vi "单个流程读取.vi"(7 "工作状态":u16, 8 "error in (no error)":errorcluster caption="错误输入（无错误）", 9 "量程":u16(ring) items=["低量程", "高量程"], 10 "测量模式":u16(ring) items=["跨度核查", "水样测量", "零点核查", "标样核查", "加标回收", "快捷测试", "空白校准", "标样校准"], 11 "测量参数":u16(ring) items=["总氮"=2, "总磷"=1, "氨氮"=3, "COD"=22]) -> (0 "error out":errorcluster, 3 "数组 2":T1(array[cluster]) {"port" format="%08x"})   [LabVIEW 2016, in "斯坦道氟化物.lvlib"]
uses:
  <vilib>/Plasmionique/MB Master/MB Master.lvlib
panel:
  out "数值":i32
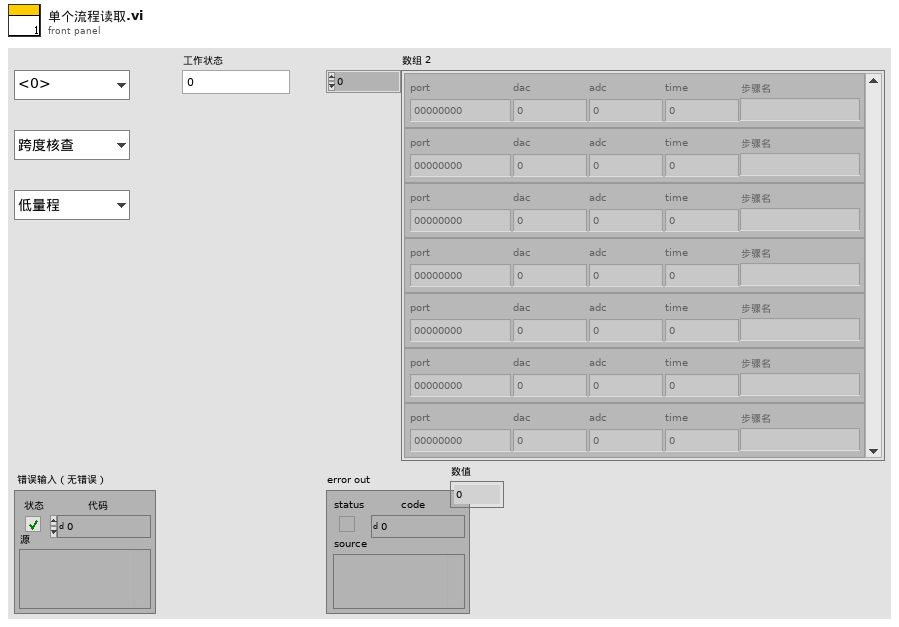
[diagram p1: front panel]
types:
  T1 = cluster{"port":i32, "dac":u8, "adc":u8, "time":u16, "步骤名":string}[]
  T2 = cluster{"port":i32, "dac":u8, "adc":u8, "time":u16, "步骤名":string}
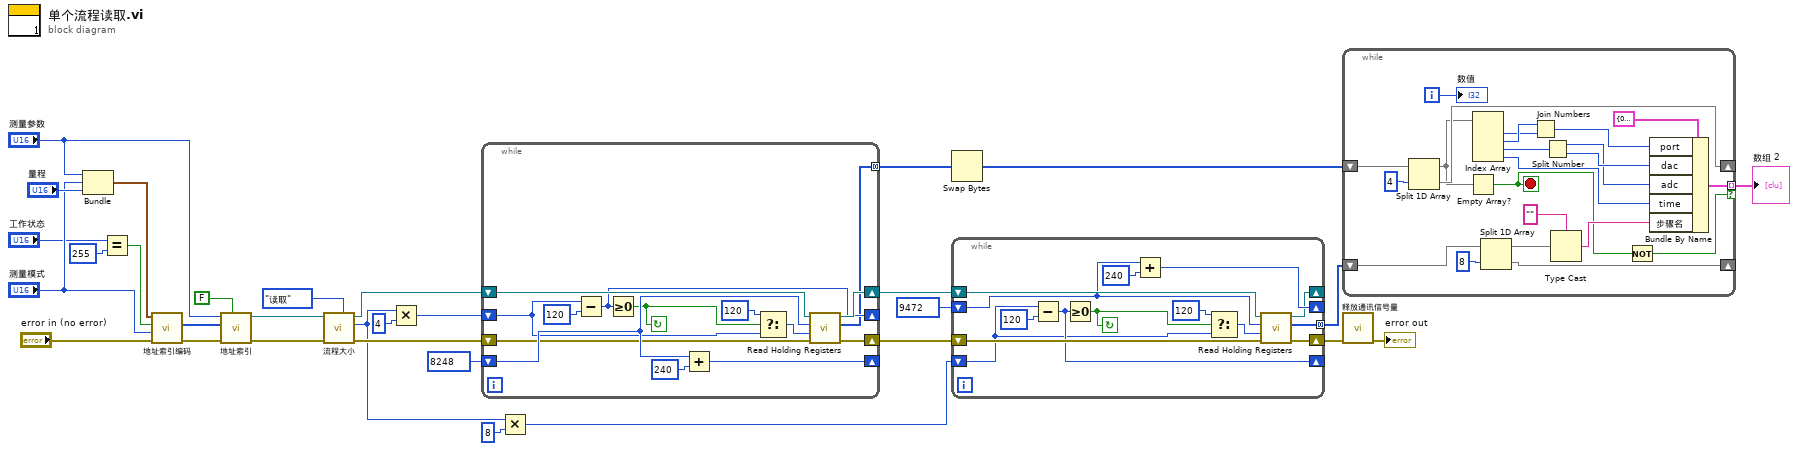
[diagram p0: block diagram]
diagram:
  n1 = Bundle("测量参数"="测量参数", "测量模式"="测量模式", "量程"="量程") -> (w26:cluster{"测量参数":u16, "测量模式":u16, "量程":u16})  [unwired: 1 in]
  n2 = Equal?(x="工作状态", y=255) -> (x = y?=w2:bool)
  n3 = call "地址索引编码.vi"("error in (no error)"="error in (no error)", "简易流程Id"="测量模式", "是否是简易流程"=w2, "参数簇"=w26) -> ("error out"=w24:errorcluster, "数组"=w25:u16[])  [unwired: 6 in]
  n4 = call "地址索引.vi"("4.2写公式？"=FALSE ("写流程？"), "error in (no error)"=w24, "values"=w25, "测量参数"="测量参数") -> ("error out"=w30:errorcluster, "MB session out"=w29:refnum<class "MB_Master.lvclass">)  [unwired: 6 in]
  n5 = call "流程大小.vi"("功能"=enum16{"写入", "读取"}."读取", "error in (no error)"=w30, "MB session in"=w29) -> ("error out"=w11:errorcluster, "大小读取"=w9:i32, "MB session out"=w10:refnum<class "MB_Master.lvclass">)  [unwired: 6 in]
  n6 = Multiply(x=w9, y=4) -> (x*y=w22:i32)
  n7 = while {
    shift-right: [w44] -> _
    shift-left: u16 8248 ("starting address") -> [w41]
    shift-right: [w43] -> w17
    shift-left: w10 -> [w42]
    shift-right: [w40] -> w16
    shift-left: w11 -> [w39]
    shift-right: [w37] -> _
    shift-left: w22 -> [w36]
    tunnel: [w32] -> w14 mode=concatenating
    stop <- w34 continue-if-true
    n8 = Subtract(x=w36, y=120) -> (x-y=w37:i32)
    n9 = Greater Or Equal To 0?(x=w37) -> (x >= 0?=w34:bool)
    n10 = Add(x=w41, y=u16 240) -> (x+y=w44:u16)
    n11 = Select(t=120 ("y"), s=w34, f=w36) -> (s? t:f=w33:i32)
    n12 = call <vilib>:"Read Holding Registers.vi"("error in (no error)"=w39, "quantity"=w33, "starting address"=w41, "MB session in"=w42) -> ("error out"=w40:errorcluster, "Registers"=w32:u16[], "MB session out"=w43:refnum<class "MB_Master.lvclass">)  [unwired: 5 in]
  }
  n13 = Multiply(x=w9, y=8) -> (x*y=w19:i32)
  n14 = Swap Bytes(anything=w14) -> (byte swapped=w13:u16[])
  n15 = while {
    shift-right: [w58] -> _
    shift-left: u16 9472 ("starting address") -> [w55]
    shift-right: [w57] -> _
    shift-left: w17 -> [w56]
    shift-right: [w54] -> w7
    shift-left: w16 -> [w53]
    shift-right: [w51] -> _
    shift-left: w19 -> [w50]
    tunnel: [w46] -> w15 mode=concatenating
    stop <- w48 continue-if-true
    n16 = Subtract(x=w50, y=120) -> (x-y=w51:i32)
    n17 = Greater Or Equal To 0?(x=w51) -> (x >= 0?=w48:bool)
    n18 = Add(x=w55, y=u16 240) -> (x+y=w58:u16)
    n19 = Select(t=120 ("y"), s=w48, f=w50) -> (s? t:f=w47:i32)
    n20 = call <vilib>:"Read Holding Registers.vi"("error in (no error)"=w53, "quantity"=w47, "starting address"=w55, "MB session in"=w56) -> ("error out"=w54:errorcluster, "Registers"=w46:u16[], "MB session out"=w57:refnum<class "MB_Master.lvclass">)  [unwired: 5 in]
  }
  n21 = while {
    shift-right: [w60] -> _
    shift-left: w15 -> [w79]
    shift-right: [w63] -> _
    shift-left: w13 -> [w81]
    tunnel: [w67] -> w12 mode=indexing if=w65
    i -> [w64]
    stop <- w66 stop-if-true
    n22 = Split 1D Array(array=w81, index=4 ("索引")) -> (first subarray=w62:u16[], second subarray=w63:u16[])
    n23 = Empty Array?(array=w62) -> (empty?=w66:bool)
    n24 = Index Array(array=w62) -> (element #1=w69:u16, element #2=w70:u16, element #3=w73:u16, element #4=w74:u16)  [unwired: 4 in]
    n25 = Split 1D Array(array=w79, index=8 ("索引")) -> (first subarray=w61:u16[], second subarray=w60:u16[])
    n26 = Join Numbers(hi=w70, lo=w69) -> ((hi.lo)=w68:u32)
    n27 = Split Number(x=w73) -> (hi(x)=w71:u8, lo(x)=w72:u8)
    n28 = Type Cast(type="", x=w61) -> (*(type *) &x=w75:string)
    n29 = Not(x=w66) -> (.not. x?=w65:bool)
    n30 = Bundle By Name(cluster=T2 {"port"=0, "dac"=0, "adc"=0, "time"=0, "步骤名"=""} ("簇 2"), "port"=w68, "dac"=w72, "adc"=w71, "time"=w74, "步骤名"=w75) -> (w67:T2)
    "数值" <- w64
  }
  "数组 2" <- w12
  n31 = call "释放通讯信号量.vi"("error in (no error)"=w7) -> ("error out"=→"error out":errorcluster)  [unwired: 10 in]
